vi "Get Character Size.vi"(8 "error in (no error)":errorcluster, 11 "Terminal in":refnum<class "Terminal.lvclass">) -> (0 "error out":errorcluster, 2 "Character Size":cluster{"Width":i16, "Height":i16}, 3 "Terminal out":refnum<class "Terminal.lvclass">)   [LabVIEW 2020, in "Terminal.lvlib" / "Terminal.lvclass"]
uses:
  Terminal.lvclass
  Terminal.lvclass/Terminal.ctl
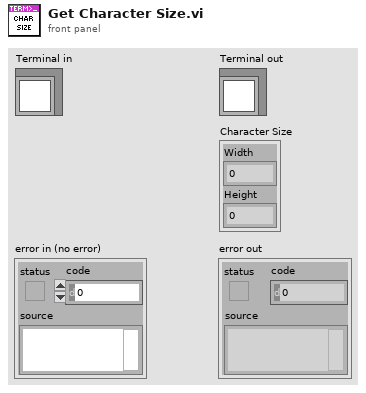
[diagram p1: front panel]
types:
  T1 = typedef "Terminal.lvlib/Terminal.lvclass/Ref Data.ctl" = cluster{"Connection":refnum<class "Connection.lvclass">, "Read Loop Running":bool, "Parse State":T2, "Terminal Options":T8, "Font Metrics":T11, "Scroll":i32, "Close Read Loop":bool, "Buffer":T7, "Pause Read Loop":bool}
  T2 = typedef "Terminal.lvlib/Terminal.lvclass/Parse State.ctl" = cluster{"Buffer State":T3, "Cursor":T4, "Attributes":T6, "Active Buffer":T7}
  T3 = typedef "Terminal.lvlib/Terminal.lvclass/Buffer State.ctl" = cluster{"Sequence":string, "ESC":bool, "Alt Buf":bool}
  T4 = typedef "Terminal.lvlib/Terminal.lvclass/Cursor.ctl" = cluster{"Cur":T5, "Saved":T5}
  T5 = typedef "Terminal.lvlib/Terminal.lvclass/Position.ctl" = cluster{"Row":i32, "Col":i32}
  T6 = typedef "Terminal.lvlib/Text Attributes.ctl" = cluster{"FG":u32, "BG":u32, "Bold":bool, "Italic":bool, "Underline":bool, "Strike":bool, "Inverse":bool}
  T7 = typedef "Terminal.lvlib/Buffer.ctl" = enum16{"Primary", "Alternate"}
  T8 = typedef "Terminal.lvlib/Terminal Options.ctl" = cluster{"Implied CR with LF":bool, "Local Echo":bool, "Tab Width":i32, "Color Scheme":T9, "Default FG":T10, "Default BG":T10, "History Length":i32, "Font Face":string, "Font Size":i16, "Rows":i32, "Cols":i32}
  T9 = typedef "Terminal.lvlib/Color Scheme.ctl" = cluster{"Black":u32, "Red":u32, "Green":u32, "Yellow":u32, "Blue":u32, "Magenta":u32, "Cyan":u32, "White":u32, "Bright Black":u32, "Bright Red":u32, "Bright Green":u32, "Bright Yellow":u32, "Bright Blue":u32, "Bright Magenta":u32, "Bright Cyan":u32, "Bright White":u32}
  T10 = typedef "Terminal.lvlib/Color.ctl" = i8
  T11 = typedef "Terminal.lvlib/Terminal.lvclass/Font Metrics.ctl" = cluster{"Width":i16, "Height":i16}
  T12 = enum16{"User-specified Font", "Application Font", "System Font", "Dialog Font"}
  T13 = cluster{"Font Name:":string, "Size":i16, "Strikeout?":bool, "Italic?":bool, "Underline?":bool, "Outline?":bool, "Shadow?":bool, "Bold?":bool}
  T14 = cluster{"left":i16, "top":i16, "right":i16, "bottom":i16}
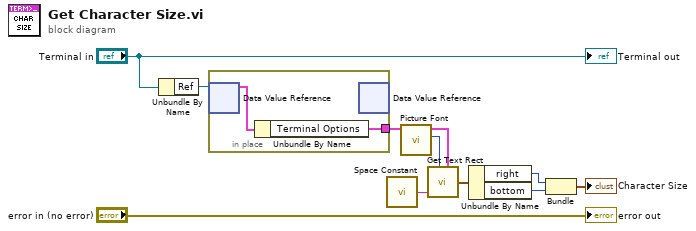
[diagram p0: block diagram]
diagram:
  n1 = Unbundle By Name("Terminal in") -> ("Ref"=w10:refnum<data-value>)
  n2 = in-place {
    in-place-border: [w12] -> w9
    n3 = in-place-dvr #1(w10) -> (w13:T1)  [unwired: 1 out]
    n4 = Unbundle By Name(w13) -> ("Terminal Options"=w12:T8)
    n5 = in-place-dvr #1() -> ()  [unwired: 1 in, 2 out]
  }
  n6 = call <vilib>:"Space Constant.vi"() -> ("String"=w6:string)
  n7 = call "Picture Font.vi"("Terminal Options"=w9) -> ("desired font"=w7:T12, "Picture Font"=w8:T13)  [unwired: 7 in, 2 out]
  n8 = call <vilib>:"Get Text Rect.vi"("desired font(Application)"=w7, "text"=w6, "[user-specified font]"=w8) -> ("rect"=w5:T14)  [unwired: 6 in]
  n9 = Unbundle By Name(w5) -> ("right"=w3:i16, "bottom"=w4:i16)
  n10 = Bundle("right"=w3, "bottom"=w4) -> (→"Character Size":cluster{"right":i16, "bottom":i16})  [unwired: 1 in]
  "error out" <- "error in (no error)"
  "Terminal out" <- "Terminal in"
